vi "S2C_IMAGE_Proc_Commands.vi"(8 "Error In":errorcluster, 11 "Settings":T1) -> (0 "Error Out":errorcluster, 2 "Stop?":bool, 3 "Response":variant)   [LabVIEW 2015]
panel:
  in  "Q-Ref":refnum<queue>
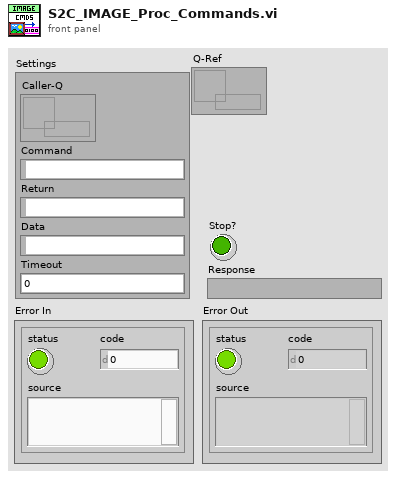
[diagram p1: front panel]
types:
  T1 = cluster{"Caller-Q":refnum<queue>, "Command":string, "Return":string, "Data":variant, "Timeout":dbl}
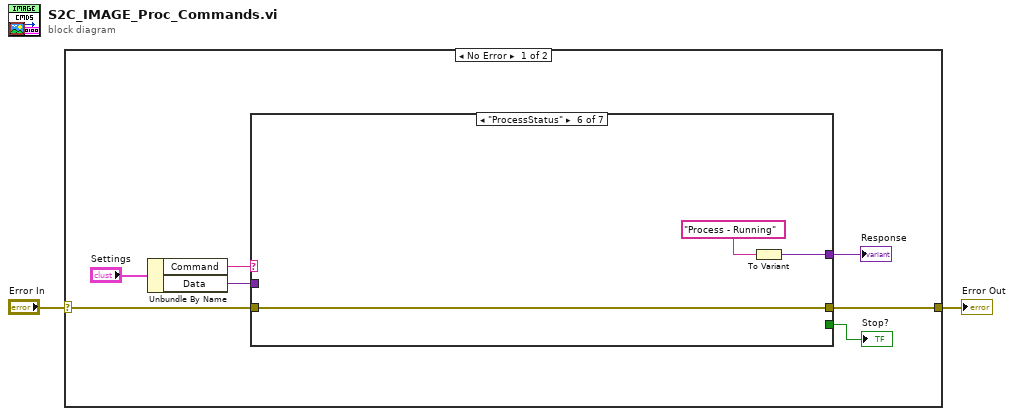
[diagram p0: block diagram]
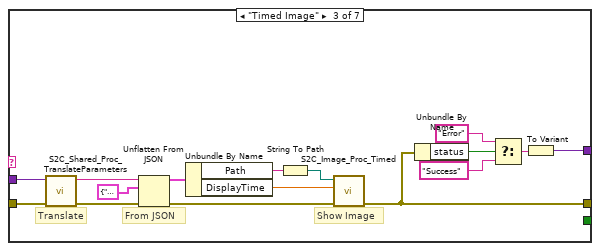
[diagram p4: hidden frame]
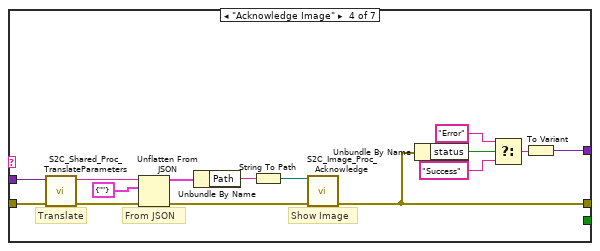
[diagram p5: hidden frame]
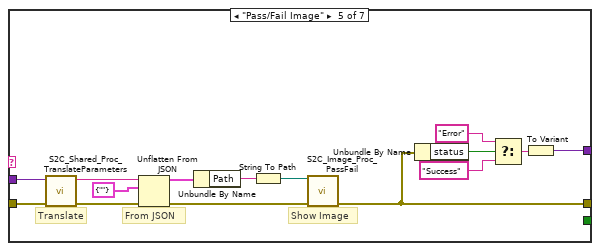
[diagram p6: hidden frame]
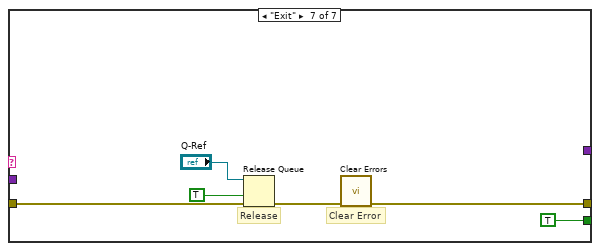
[diagram p7: hidden frame]
diagram:
  n1 = case shown="No Error" "Error In" {
    selector: "Error In" -> [w7 w67]
    tunnel: [w6 w67] -> w1
    frame No Error {
      n2 = Unbundle By Name("Settings") -> ("Command"=w8:string, "Data"=w9:variant)
      n3 = case shown="\"ProcessStatus\"" w8 {
        tunnel: w7 -> [w10 w11 w18 w33 w48 w60 w66]
        tunnel: w9 -> [_ _ w17 w32 w47 _ _]
        tunnel: [w10 w11 w23 w38 w53 w60 w61] -> w6
        tunnel: [_ _ w27 w42 w57 w59 _] -> w4
        tunnel: [_ _ _ _ _ _ TRUE] -> w3
        frame "Other", Default {
        }
        frame "Init" {
        }
        frame "Timed Image" {
          # "Show Image"
          # "Translate"
          # "From JSON"
          n4 = call "S2C_Shared_Proc_TranslateParameters.vi"("Error In"=w18, "Data"=w17) -> ("Error Out"=w20:errorcluster, "JSON Cluster"=w21:string)  [unwired: 8 in]
          n5 = Unflatten From JSON(JSON string=w21, type and defaults=cluster{"Path":string, "DisplayTime":dbl} {"Path"="", "DisplayTime"=0.0}, error in (no error)=w20) -> (value=w19:cluster{"Path":string, "DisplayTime":dbl}, error out=w12:errorcluster)  [unwired: 4 in]
          n6 = Unbundle By Name(w19) -> ("Path"=w14:string, "DisplayTime"=w15:dbl)
          n7 = String To Path(string=w14) -> (path=w13:path)
          n8 = call "S2C_Image_Proc_Timed.vi"("Error In"=w12, "DisplayTime"=w15, "ImagePath"=w13) -> ("Error Out"=w23:errorcluster)  [unwired: 8 in]
          n9 = Unbundle By Name(w23) -> ("status"=w22:bool)
          n10 = Select(t="Error", s=w22, f="Success") -> (s? t:f=w24:string)
          n11 = To Variant(anything=w24) -> (Variant=w27:variant)
        }
        frame "Acknowledge Image" {
          # "Show Image"
          # "Translate"
          # "From JSON"
          n12 = call "S2C_Shared_Proc_TranslateParameters.vi"("Error In"=w33, "Data"=w32) -> ("Error Out"=w35:errorcluster, "JSON Cluster"=w36:string)  [unwired: 8 in]
          n13 = Unflatten From JSON(JSON string=w36, type and defaults=cluster{"Path":string} {"Path"=""}, error in (no error)=w35) -> (value=w34:cluster{"Path":string}, error out=w28:errorcluster)  [unwired: 4 in]
          n14 = Unbundle By Name(w34) -> ("Path"=w30:string)
          n15 = String To Path(string=w30) -> (path=w29:path)
          n16 = call "S2C_Image_Proc_Acknowledge.vi"("Error In"=w28, "ImagePath"=w29) -> ("Error Out"=w38:errorcluster)  [unwired: 9 in]
          n17 = Unbundle By Name(w38) -> ("status"=w37:bool)
          n18 = Select(t="Error", s=w37, f="Success") -> (s? t:f=w39:string)
          n19 = To Variant(anything=w39) -> (Variant=w42:variant)
        }
        frame "Pass/Fail Image" {
          # "Show Image"
          # "Translate"
          # "From JSON"
          n20 = call "S2C_Shared_Proc_TranslateParameters.vi"("Error In"=w48, "Data"=w47) -> ("Error Out"=w50:errorcluster, "JSON Cluster"=w51:string)  [unwired: 8 in]
          n21 = Unflatten From JSON(JSON string=w51, type and defaults=cluster{"Path":string} {"Path"=""}, error in (no error)=w50) -> (value=w49:cluster{"Path":string}, error out=w43:errorcluster)  [unwired: 4 in]
          n22 = Unbundle By Name(w49) -> ("Path"=w45:string)
          n23 = String To Path(string=w45) -> (path=w44:path)
          n24 = call "S2C_Image_Proc_PassFail.vi"("Error In"=w43, "ImagePath"=w44) -> ("Error Out"=w53:errorcluster)  [unwired: 8 in, 1 out]
          n25 = Unbundle By Name(w53) -> ("status"=w52:bool)
          n26 = Select(t="Error", s=w52, f="Success") -> (s? t:f=w54:string)
          n27 = To Variant(anything=w54) -> (Variant=w57:variant)
        }
        frame "ProcessStatus" {
          n28 = To Variant(anything="Process - Running") -> (Variant=w59:variant)
        }
        frame "Exit" {
          # "Clear Error"
          # "Release"
          n29 = Release Queue(queue="Q-Ref", force destroy? (F)=TRUE, error in (no error)=w66) -> (error out=w64:errorcluster)  [unwired: 2 out]
          n30 = call <vilib>:"Clear Errors.vi"("error in (no error)"=w64) -> ("error out"=w61:errorcluster)  [unwired: 5 in, 1 out]
        }
      }
      "Response" <- w4
      "Stop?" <- w3
    }
    frame Error {
    }
  }
  "Error Out" <- w1
